vi "读取画笔.vi"(8 "error in (no error)":errorcluster caption="错误输入（无错误）", 11 "图形输入":refnum<class "图形.lvclass">) -> (0 "error out":errorcluster caption="错误输出", 2 "画笔":T1={"Width"=1, "Style"=enum."Solid"}, 3 "图形输出":refnum<class "图形.lvclass">)   [LabVIEW 2011, in "图形.lvclass"]
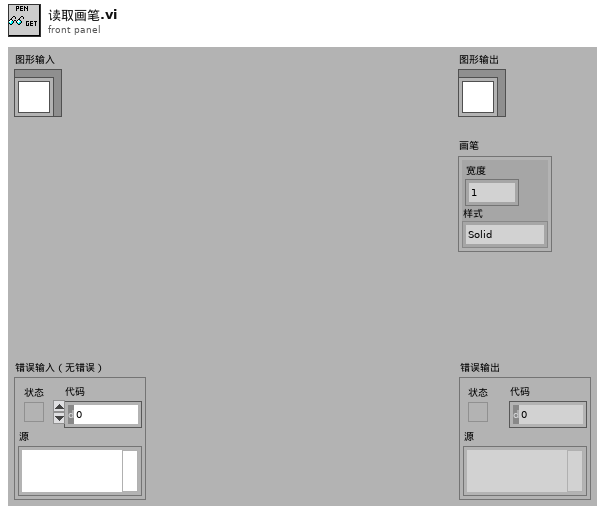
[diagram p1: front panel]
types:
  T1 = cluster{"Width":u16, "Style":enum32{"Solid", "Dash", "Dot", "DashDot", "DashDotDot"}}
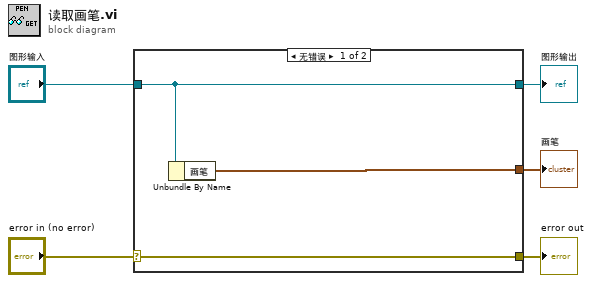
[diagram p0: block diagram]
diagram:
  n1 = case shown="无错误" "error in (no error)" {
    selector: "error in (no error)" -> [w8 w9]
    tunnel: [w8 w9] -> w4
    tunnel: [w7 w10] -> w2
    tunnel: "图形输入" -> [w7 w10]
    tunnel: [w6 _] -> w1
    frame No Error {
      n2 = Unbundle By Name(w7) -> ("画笔"=w6:T1)
    }
    frame Error {
    }
  }
  "error out" <- w4
  "图形输出" <- w2
  "画笔" <- w1
